vi "ControlSub.vi"(0 "AxisForceSample":dbl[](array[numeric]), 1 "Command":dbl[](array[numeric]), 3 "Angel":bool[](array[boolean]), 4 "AngleSample":dbl[](array[numeric]), 5 "TorqueSample":dbl[](array[numeric]), 6 "Torque":bool[](array[boolean]), 7 "TempAnIn":dbl[](array[numeric]), 8 "syn-error":dbl[](array[numeric]), 11 "ChannelSetArray":T1[](array[typedef]) {"Enable" items=["不使能", "使能"]; "Wave" items=["0指令", "正弦波", "方波", "三角波", "常值", "波形数据", "白噪声", "正弦扫频", "梯度加载", "VMIC"]; "ChannelType" items=["标准波形跟踪"=1, "扫频测试"=2, "消除多余力"=3, "梯度加载"=4, "载荷谱跟踪"=5, "模拟输入跟踪"=9]; "ChannelStatus" items=["通道关", "位置通道", "加载通道"]}, 12 "ControlPara":dbl[][](array[numeric])) -> (9 "syn out":dbl[](array[numeric]), 10 "diff syn out 2":dbl[](array[numeric]), 14 "ControlOutput":dbl[](array[numeric]), 15 "Forward":dbl[](array[numeric]), 17 "TempAnOut":dbl[](array[numeric]), 18 "control out":dbl[](array[numeric]), 19 "Commandout":dbl[](array[numeric]))   [LabVIEW 2014]
uses:
  ChannelCommand.ctl
  Control 1.ctl
  WaveType.ctl
  MoterEnable.ctl
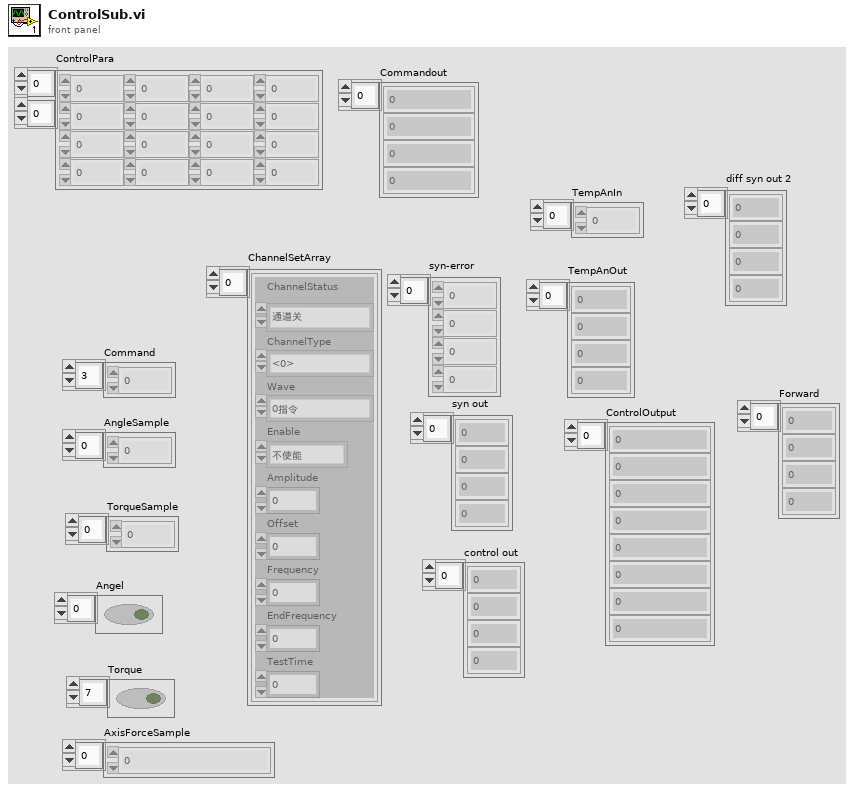
[diagram p1: front panel]
types:
  T1 = typedef "ChannelCommand.ctl" = cluster{"ChannelStatus":T2, "ChannelType":i32, "Wave":T3, "Enable":T4, "Amplitude":dbl, "Offset":dbl, "Frequency":dbl, "EndFrequency":dbl, "TestTime":dbl}
  T2 = typedef "Control 1.ctl" = i32
  T3 = typedef "WaveType.ctl" = i32
  T4 = typedef "MoterEnable.ctl" = u16
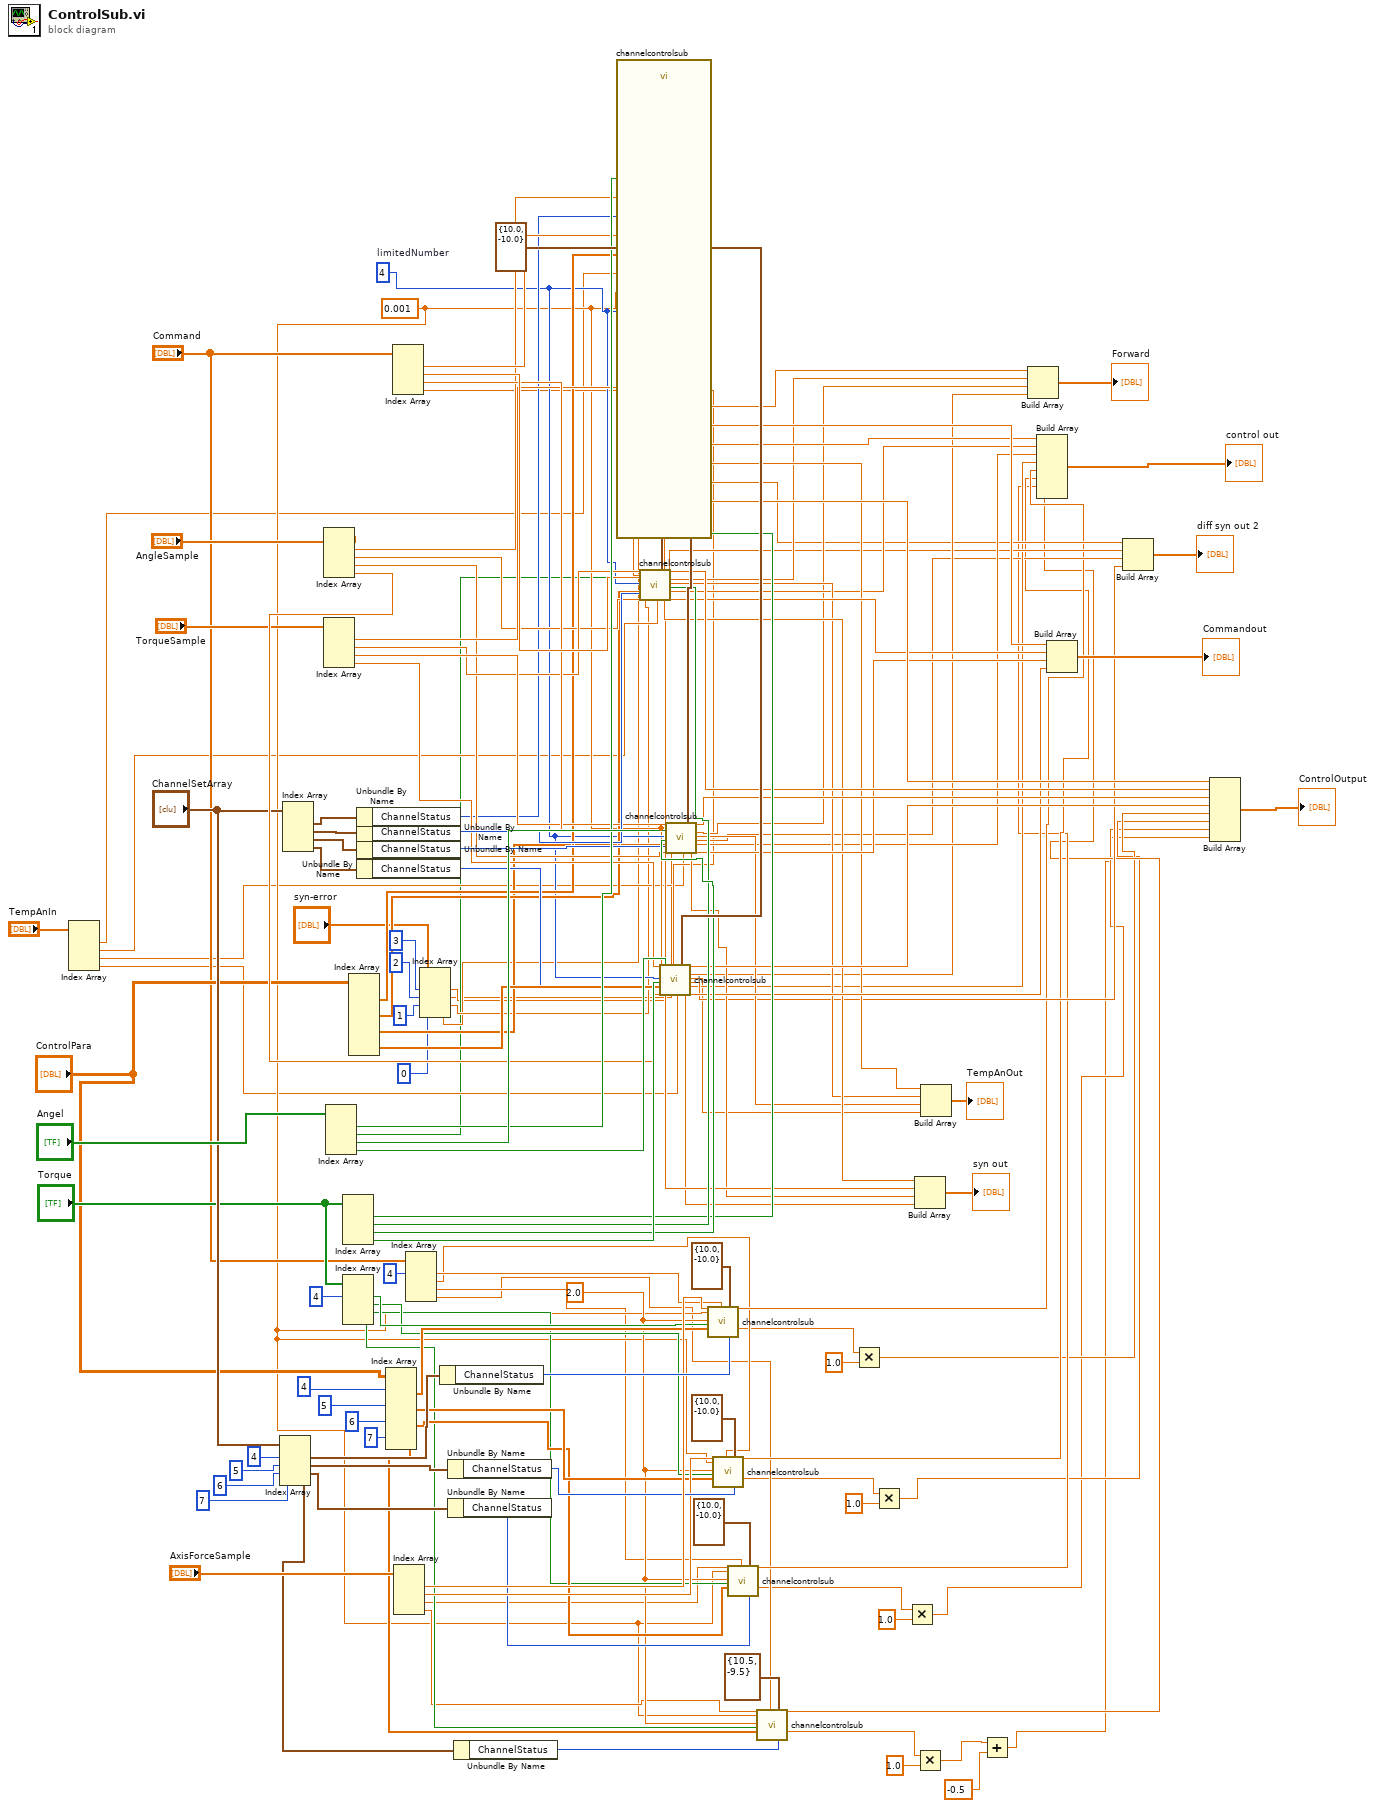
[diagram p0: block diagram]
diagram:
  w37 = 2.0 ("Limit Number")
  w32 = 0.001 ("dt")
  w95 = 4  # limitedNumber
  w144 = cluster{"output high":dbl, "output low":dbl} {"output high"=10.0, "output low"=-10.0} ("output range")
  n1 = Index Array(array="TempAnIn") -> (element #1=w10:dbl, element #2=w8:dbl, element #3=w9:dbl, element #4=w7:dbl)  [unwired: 4 in]
  n2 = Index Array(array="ChannelSetArray", index #1=4 ("索引"), index #2=5 ("索引"), index #3=6 ("索引"), index #4=7 ("索引")) -> (element #1=w67:T1, element #2=w53:T1, element #3=w44:T1, element #4=w36:T1)
  n3 = Index Array(array="ChannelSetArray") -> (element #1=w149:T1, element #2=w148:T1, element #3=w146:T1, element #4=w145:T1)  [unwired: 4 in]
  n4 = Index Array(array="AngleSample") -> (element #1=w125:dbl, element #2=w124:dbl, element #3=w123:dbl, element #4=w82:dbl)  [unwired: 4 in]
  n5 = Index Array(array="TorqueSample") -> (element #1=w126:dbl, element #2=w127:dbl, element #3=w128:dbl, element #4=w129:dbl)  [unwired: 4 in]
  n6 = Index Array(array="Angel") -> (element #1=w137:bool, element #2=w3:bool, element #3=w138:bool, element #4=w139:bool)  [unwired: 4 in]
  n7 = Index Array(array="Torque") -> (element #1=w140:bool, element #2=w141:bool, element #3=w142:bool, element #4=w143:bool)  [unwired: 4 in]
  n8 = Index Array(array="Torque", index #1=4 ("索引")) -> (element #1=w62:bool, element #2=w46:bool, element #3=w45:bool, element #4=w38:bool)  [unwired: 3 in]
  n9 = Index Array(array="ControlPara") -> (element #1=w121:dbl[], element #2=w120:dbl[], element #3=w119:dbl[], element #4=w136:dbl[])  [unwired: 8 in]
  n10 = Unbundle By Name(w149) -> ("ChannelStatus"=w122:T2)
  n11 = Unbundle By Name(w148) -> ("ChannelStatus"=w133:T2)
  n12 = Unbundle By Name(w146) -> ("ChannelStatus"=w134:T2)
  n13 = Unbundle By Name(w145) -> ("ChannelStatus"=w135:T2)
  n14 = Index Array(array="ControlPara", index (row) #1=4 ("索引"), index (row) #2=5 ("索引 (行)"), index (row) #3=6 ("索引 (行)"), index (row) #4=7 ("索引 (行)")) -> (element #1=w59:dbl[], element #2=w50:dbl[], element #3=w47:dbl[], element #4=w41:dbl[])  [unwired: 4 in]
  n15 = Index Array(array="Command") -> (element #1=w132:dbl, element #2=w131:dbl, element #3=w130:dbl, element #4=w76:dbl)  [unwired: 4 in]
  n16 = Index Array(array="AxisForceSample") -> (element #1=w65:dbl, element #2=w51:dbl, element #3=w34:dbl, element #4=w33:dbl)  [unwired: 4 in]
  n17 = Index Array(array="Command", index #1=4 ("索引")) -> (element #1=w56:dbl, element #2=w27:dbl, element #3=w26:dbl, element #4=w25:dbl)  [unwired: 3 in]
  n18 = Index Array(array="syn-error", index #1=3 ("索引"), index #2=2 ("索引"), index #3=1 ("索引"), index #4=0 ("索引")) -> (element #1=w2:dbl, element #2=w1:dbl, element #3=w5:dbl, element #4=w4:dbl)
  n19 = Unbundle By Name(w67) -> ("ChannelStatus"=w73:T2)
  n20 = Unbundle By Name(w53) -> ("ChannelStatus"=w52:T2)
  n21 = Unbundle By Name(w44) -> ("ChannelStatus"=w43:T2)
  n22 = Unbundle By Name(w36) -> ("ChannelStatus"=w35:T2)
  n23 = call "channelcontrolsub.vi"("TorqueSample"=w126, "dt"=w32, "Limit Number"=w95, "Torque"=w140, "ControlPara"=w121, "AngleSample"=w125, "Angel"=w137, "syn-Error"=w4, "Command"=w132, "TempAngle"=w10, "output range"=w144, "ChannelStatus"=w122) -> ("syn out"=w107:dbl, "output"=w115:dbl, "forward"=w93:dbl, "TempAngleOut"=w101:dbl, "diff syn out 2"=w88:dbl, "control out"=w98:dbl, "Commandout"=w113:dbl)  [unwired: 9 in]
  n24 = call "channelcontrolsub.vi"("TorqueSample"=w127, "dt"=w32, "Limit Number"=w95, "Torque"=w141, "ControlPara"=w120, "AngleSample"=w124, "Angel"=w3, "syn-Error"=w5, "Command"=w131, "TempAngle"=w8, "output range"=w144, "ChannelStatus"=w133) -> ("syn out"=w106:dbl, "output"=w116:dbl, "forward"=w92:dbl, "TempAngleOut"=w102:dbl, "diff syn out 2"=w87:dbl, "control out"=w97:dbl, "Commandout"=w112:dbl)  [unwired: 9 in]
  n25 = call "channelcontrolsub.vi"("TorqueSample"=w129, "dt"=w32, "Limit Number"=w95, "Torque"=w143, "ControlPara"=w136, "AngleSample"=w82, "Angel"=w139, "syn-Error"=w2, "Command"=w76, "TempAngle"=w7, "output range"=w144, "ChannelStatus"=w135) -> ("syn out"=w104:dbl, "output"=w118:dbl, "forward"=w90:dbl, "TempAngleOut"=w84:dbl, "diff syn out 2"=w86:dbl, "control out"=w85:dbl, "Commandout"=w110:dbl)  [unwired: 9 in]
  n26 = call "channelcontrolsub.vi"("TorqueSample"=w128, "dt"=w32, "Limit Number"=w95, "Torque"=w142, "ControlPara"=w119, "AngleSample"=w123, "Angel"=w138, "syn-Error"=w1, "Command"=w130, "TempAngle"=w9, "output range"=w144, "ChannelStatus"=w134) -> ("syn out"=w105:dbl, "output"=w117:dbl, "forward"=w91:dbl, "TempAngleOut"=w103:dbl, "diff syn out 2"=w83:dbl, "control out"=w96:dbl, "Commandout"=w111:dbl)  [unwired: 9 in]
  n27 = call "channelcontrolsub.vi"("TorqueSample"=w65, "dt"=w32, "Limit Number"=w37, "Torque"=w62, "ControlPara"=w59, "Command"=w56, "output range"=cluster{"output high":dbl, "output low":dbl} {"output high"=10.0, "output low"=-10.0}, "ChannelStatus"=w73) -> ("output"=w31:dbl, "control out"=w24:dbl)  [unwired: 13 in, 5 out]
  n28 = call "channelcontrolsub.vi"("TorqueSample"=w51, "dt"=w32, "Limit Number"=w37, "Torque"=w46, "ControlPara"=w50, "Command"=w27, "output range"=cluster{"output high":dbl, "output low":dbl} {"output high"=10.0, "output low"=-10.0}, "ChannelStatus"=w52) -> ("output"=w30:dbl, "control out"=w21:dbl)  [unwired: 13 in, 5 out]
  n29 = call "channelcontrolsub.vi"("TorqueSample"=w34, "dt"=w32, "Limit Number"=w37, "Torque"=w45, "ControlPara"=w47, "Command"=w26, "output range"=cluster{"output high":dbl, "output low":dbl} {"output high"=10.0, "output low"=-10.0}, "ChannelStatus"=w43) -> ("output"=w29:dbl, "control out"=w17:dbl)  [unwired: 13 in, 5 out]
  n30 = call "channelcontrolsub.vi"("TorqueSample"=w33, "dt"=w32, "Limit Number"=w37, "Torque"=w38, "ControlPara"=w41, "Command"=w25, "output range"=cluster{"output high":dbl, "output low":dbl} {"output high"=10.5, "output low"=-9.5}, "ChannelStatus"=w35) -> ("output"=w28:dbl, "control out"=w14:dbl)  [unwired: 13 in, 5 out]
  n31 = Multiply(x=w24, y=1.0) -> (x*y=w22:dbl)
  n32 = Multiply(x=w21, y=1.0) -> (x*y=w20:dbl)
  n33 = Multiply(x=w17, y=1.0) -> (x*y=w16:dbl)
  n34 = Build Array(w107, w106, w105, w104) -> (→"syn out":dbl[])
  n35 = Multiply(x=w14, y=1.0) -> (x*y=w13:dbl)
  n36 = Build Array(w101, w102, w103, w84) -> (→"TempAnOut":dbl[])
  n37 = Add(x=w13, y=-0.5) -> (x+y=w11:dbl)
  n38 = Build Array(w93, w92, w91, w90) -> (→"Forward":dbl[])
  n39 = Build Array(w98, w97, w96, w85, w31, w30, w29, w28) -> (→"control out":dbl[])
  n40 = Build Array(w113, w112, w111, w110) -> (→"Commandout":dbl[])
  n41 = Build Array(w88, w87, w83, w86) -> (→"diff syn out 2":dbl[])
  n42 = Build Array(w115, w116, w117, w118, w22, w20, w16, w11) -> (→"ControlOutput":dbl[])
